vi "AnguloFenda.vi"() -> (0 "AngFenda":dbl)   [LabVIEW 2018]
uses:
  Global_Telescopio.vi
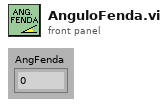
[diagram p1: front panel]
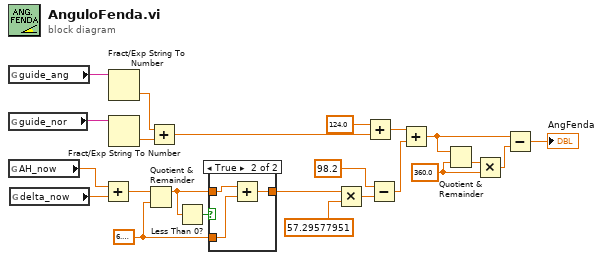
[diagram p0: block diagram]
diagram:
  w7 = 360.0
  w12 = 6.283185307179586
  n1 = global read "Global_Telescopio.vi" "guide_ang"() -> (w22:string)
  n2 = global read "Global_Telescopio.vi" "guide_nor"() -> (w23:string)
  n3 = global read "Global_Telescopio.vi" "AH_now"() -> (w19:dbl)
  n4 = global read "Global_Telescopio.vi" "delta_now"() -> (w20:dbl)
  n5 = Add(x=w19, y=w20) -> (x+y=w11:dbl)
  n6 = Fract/Exp String To Number(string=w22) -> (number=w18:dbl)  [unwired: 3 in, 1 out]
  n7 = Fract/Exp String To Number(string=w23) -> (number=w21:dbl)  [unwired: 3 in, 1 out]
  n8 = Quotient & Remainder(x=w11, y=w12) -> (x-y*floor(x/y)=w14:dbl)  [unwired: 1 out]
  n9 = Add(x=w18, y=w21) -> (x+y=w2:dbl)
  n10 = Less Than 0?(x=w14) -> (x < 0?=w16:bool)
  n11 = case shown="True" w16 {
    tunnel: w14 -> [w24 w27]
    tunnel: [w24 w25] -> w13
    tunnel: w12 -> [_ w26]
    frame False {
    }
    frame True {
      n12 = Add(x=w27, y=w26) -> (x+y=w25:dbl)
    }
  }
  n13 = Multiply(x=w13, y=57.29577951 ("x*y")) -> (x*y=w10:dbl)
  n14 = Add(x=124.0, y=w2) -> (x+y=w3:dbl)
  n15 = Subtract(x=98.2, y=w10) -> (x-y=w9:dbl)
  n16 = Add(x=w3, y=w9) -> (x+y=w6:dbl)
  n17 = Quotient & Remainder(x=w6, y=w7) -> (floor(x/y)=w8:dbl)  [unwired: 1 out]
  n18 = Multiply(x=w8, y=w7) -> (x*y=w5:dbl)
  n19 = Subtract(x=w6, y=w5) -> (x-y=→"AngFenda":dbl)
